vi "TextControlledInstrumWriteCommands.vi"(8 "error in (no error)":errorcluster, 9 "timeout in ms (100)":i32=100, 10 "Multi-line String":string, 11 "IO Queue":refnum<queue>) -> (0 "error out":errorcluster, 1 "timed out?":bool)   [LabVIEW 2019]
uses:
  TextControlledInstrumIOQueuePacket.ctl
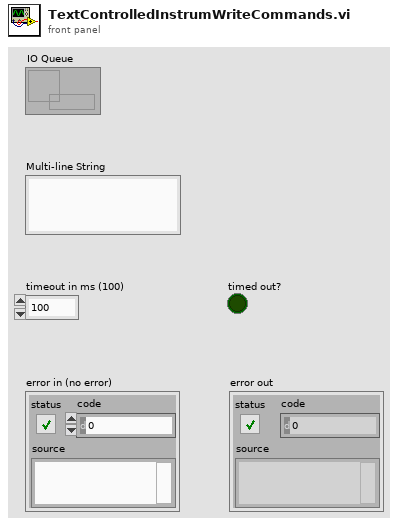
[diagram p1: front panel]
types:
  T1 = typedef "TextControlledInstrumIOQueuePacket.ctl" = cluster{"Operation":enum16{"read", "write", "reserved2", "reserved3", "reserved4", "reserved5", "reserved6", "reserved7"}, "Data":string, "Queue":refnum<queue>}
  T2 = enum16{"read", "write", "reserved2", "reserved3", "reserved4", "reserved5", "reserved6", "reserved7"}
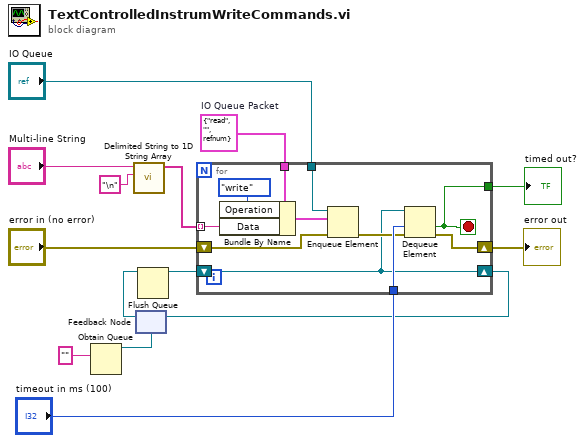
[diagram p0: block diagram]
diagram:
  w8 = T1 {"Operation"=enum."read", "Data"="", "Queue"=refnum}  # IO Queue Packet
  n1 = Obtain Queue(element data type="") -> (queue out=w6:refnum<queue>)  [unwired: 4 in, 2 out]
  n2 = call <vilib>:"Delimited String to 1D String Array.vi"("delimiter"="\n", "delimited string"="Multi-line String") -> ("string array"=w14:string[])  [unwired: 9 in]
  n3 = feedback #1(w6) -> (w5:refnum<queue>)
  n4 = Flush Queue(queue=w5) -> (queue out=w3:refnum<queue>)  [unwired: 1 in, 2 out]
  n5 = for {
    shift-right: [w17] -> w11
    shift-left: "error in (no error)" -> [w24]
    tunnel: "IO Queue" -> [w22]
    tunnel: w14 -> [w21] mode=indexing
    tunnel: w8 -> [w20]
    tunnel: "timeout in ms (100)" -> [w19]
    tunnel: [w16] -> w2
    shift-right: [w15] -> w1
    shift-left: w3 -> [w15]
    stop <- w16 stop-if-true
    n6 = Bundle By Name(cluster=w20, "Operation"=T2."write", "Data"=w21) -> (w25:T1)
    n7 = Enqueue Element(queue=w22, element=w25, error in (no error)=w24) -> (error out=w18:errorcluster)  [unwired: 1 in, 2 out]
    n8 = Dequeue Element(queue=w15, timeout in ms (-1)=w19, error in (no error)=w18) -> (timed out?=w16:bool, error out=w17:errorcluster)  [unwired: 2 out]
  }
  "error out" <- w11
  "timed out?" <- w2
  n9 = feedback-in #1(w1) -> ()
